vi "toml_example_datetime.vi"() -> ()   [LabVIEW 2017]
panel:
  out "time stamp":timestamp format="%<%Y-%02m-%02dT%H:%M:%S%6u>T"
  out "error out":errorcluster
  out "time stamp 2":timestamp format="%<%Y-%02m-%02dT%H:%M:%S%6u>T"
  out "error out 2":errorcluster
  out "time stamp 3":timestamp format="%<%Y-%02m-%02dT%H:%M:%S%6u>T"
  out "error out 3":errorcluster
  out "date/time string 3":string
  out "date/time string 2":string
  out "date/time string":string
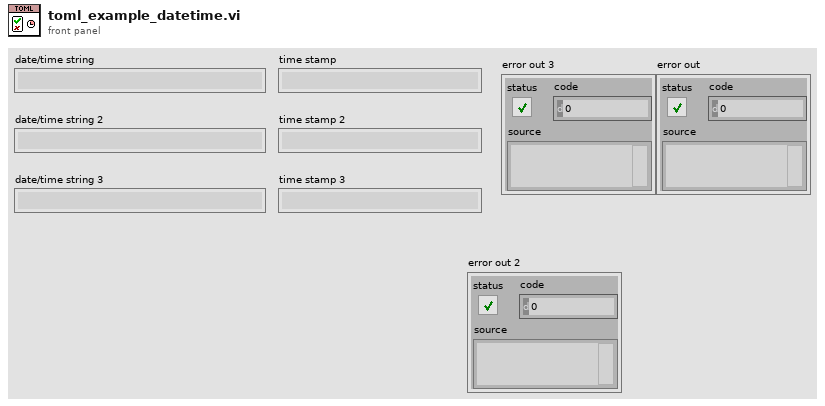
[diagram p1: front panel]
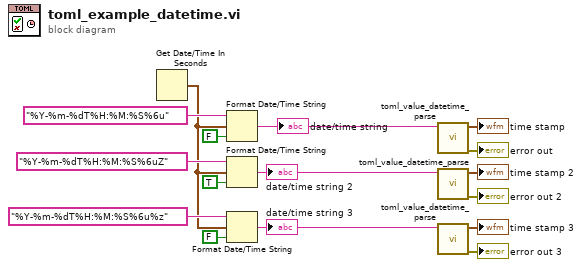
[diagram p0: block diagram]
diagram:
  n1 = Get Date/Time In Seconds() -> (seconds since 1Jan1904=w10:timestamp)
  n2 = Format Date/Time String(time format string (%c)="%Y-%m-%dT%H:%M:%S%6u", seconds (now)=w10, UTC format=FALSE) -> (date/time string=w9:string)
  "date/time string" <- w9
  n3 = Format Date/Time String(time format string (%c)="%Y-%m-%dT%H:%M:%S%6uZ", seconds (now)=w10, UTC format=TRUE) -> (date/time string=w8:string)
  "date/time string 2" <- w8
  n4 = Format Date/Time String(time format string (%c)="%Y-%m-%dT%H:%M:%S%6u%z", seconds (now)=w10, UTC format=FALSE) -> (date/time string=w7:string)
  "date/time string 3" <- w7
  n5 = call "toml_value_datetime_parse.vi"("value"=w9) -> ("error out"=→"error out":errorcluster, "time stamp"=→"time stamp":timestamp)  [unwired: 9 in]
  n6 = call "toml_value_datetime_parse.vi"("value"=w8) -> ("error out"=→"error out 2":errorcluster, "time stamp"=→"time stamp 2":timestamp)  [unwired: 9 in]
  n7 = call "toml_value_datetime_parse.vi"("value"=w7) -> ("error out"=→"error out 3":errorcluster, "time stamp"=→"time stamp 3":timestamp)  [unwired: 9 in]
